vi "configuration UI.vi"() -> ()   [LabVIEW 2015, in "TDMS datalogger editor node.lvclass"]
uses:
  TDMS datalogger editor node.lvclass
  <vilib>/NI/Configuration Framework/Node/NodeRef.ctl
  <vilib>/NI/Configuration Framework/Node/NISE_CEF_Node.lvclass
  <vilib>/NI/AMC/Message Queue.ctl
  <vilib>/NI/AMC/Message.ctl
  <vilib>/NI/Tools/Keyed Array/KeyedArray.ctl
  <vilib>/NI/Configuration Framework/Node/UserEventRef.ctl
  <vilib>/NI/Configuration Framework/Controls/EventCluster.ctl
  <vilib>/NI/DCAF UI Toolkit/Controls/Move One Right.ctl
  <vilib>/NI/DCAF UI Toolkit/Controls/Move All Right.ctl
  <vilib>/NI/DCAF UI Toolkit/Controls/Move One Left.ctl
  <vilib>/NI/Configuration Framework/Node/NodeChangeEvent.ctl
  module/configuration/Logging Type.ctl
  module/configuration/Edge Direction.ctl
  module/configuration/Trigger Type.ctl
  module/configuration/Hidable controls.ctl
  module/configuration/TDMS datalogger configuration.lvclass
  <vilib>/Utility/miscctls.llb/LVPositionTypeDef.ctl
  TDMS datalogger editor node.lvclass/TDMS datalogger editor node.ctl
  module/configuration/TDMS datalogger configuration.lvclass/TDMS datalogger configuration.ctl
  <vilib>/NI/Tag Bus/tag/tag descriptor.lvclass/tag descriptor.ctl
  <vilib>/NI/Configuration Framework/serializable configuration/NISE_CEF_serializable configuration.lvclass/NISE_CEF_serializable configuration.ctl
  module/configuration/Write scans per write.vi
  module/configuration/Write queue size.vi
  module/configuration/Write Pre-trigger Blocks.vi
  module/configuration/Write Blocks to Log.vi
  module/configuration/Write Path.vi
  module/configuration/Write log name.vi
  module/configuration/Write backup directory.vi
  module/configuration/Read logrotate_options.vi
  module/configuration/Write logrotate_options.vi
  module/configuration/Write channel pattern matches.vi
  module/configuration/Write Logging Type.vi
  module/configuration/Write Edge Direction.vi
  module/configuration/Write Trigger Type.vi
  Write channel table.vi
  Write avail tags table.vi
  module/configuration/Read backup directory.vi
  module/configuration/Read Path.vi
  module/configuration/Read queue size.vi
  module/configuration/Read scans per write.vi
  module/configuration/Read add enable channel.vi
  module/configuration/Read channel pattern matches.vi
  module/configuration/Read log name.vi
  module/configuration/Read Trigger Type.vi
  module/configuration/Read Pre-trigger Blocks.vi
  module/configuration/Read Logging Type.vi
  module/configuration/Read Edge Direction.vi
  module/configuration/Read Blocks to Log.vi
  <vilib>/NI/DCAF/Tag Editor Core/Configuration Editor/Classes/Module editor node/Read Module Configuration.vi
  <vilib>/Utility/LVClass/Get LV Class Name.vi
  <vilib>/NI/Configuration Framework/error generator/NISE_error generator.vi
  Table Items.vi
  <vilib>/NI/Tag Bus Module Framework/module configuration/TBM module configuration.lvclass
  <vilib>/NI/Tag Bus/tag/tag descriptor.lvclass
  <vilib>/NI/DCAF/Tag Editor Core/Configuration Editor/Classes/Module editor node/module editor node.lvclass
  <vilib>/NI/Module Execution Interface/Engine Configuration/engine configuration.lvclass
  <vilib>/NI/Configuration Framework/NISE_CEF_TreeControl.lvlib
  <vilib>/NI/DCAF/Tag Editor Core/Configuration Editor/Classes/Engine Parent/Engine Parent Editor Node.lvclass
  <vilib>/NI/Configuration Framework/serializable configuration/NISE_CEF_serializable configuration.lvclass
  <vilib>/NI/DCAF UI Toolkit/Controls/DCAF UI Elements.lvlib
  <vilib>/NI/Tools/Keyed Array/Tools_KeyedArray.lvlib
  <vilib>/NI/AMC/AMC.lvlib
panel:
  in  "output cluster":T1
  in  "node change":T2
  in  "Tab Control":T3(tab)
  in  "Filter":string
  in  "channels":i32(listbox)
  in  "remove":T4
  in  "avail tags":i32(listbox)=-1
  in  "add all":T5
  in  "add1":T6
  in  "Edge Direction":T7
  out "Trigger Channel":string
  in  "Trigger Type":T8
  in  "Total Blocks to Log":i32=20
  in  "Pre-trigger Blocks":i32=20
  in  "Logging Type":T9
  out "Enable Tag":string
  in  "use enable channel":bool
  in  "queue size":u16=2
  in  "file name error":bool
  in  "Log Directory":string
  in  "File Name":string
  in  "path error":bool
  in  "recalc":bool
  out "Approximate memory usage":dbl
  in  "Block Size (scans per write)":u16=20
  in  "Log Directory":path
  in  "Maximum age of files (days)":dbl=365.0
  in  "Maximum file size (KB)":i64=10000
  in  "Rotate count":u32 caption="Maximum number of archived files to keep"
  in  "archive in place":bool caption="Archive old logs in original directory"
  in  "Archive Directory":string
  in  "Archive Directory":path
  in  "archive error":bool
  in  "Channel Subscription Pattern Matches":string[](array[string])
  in  "Enable Dynamic Mapping":bool
  in  "user event":T10
  in  "main queue":T11
  in  "node ref":T12
  # "Note: This value ignores dynamic mapping"
  # "kB"
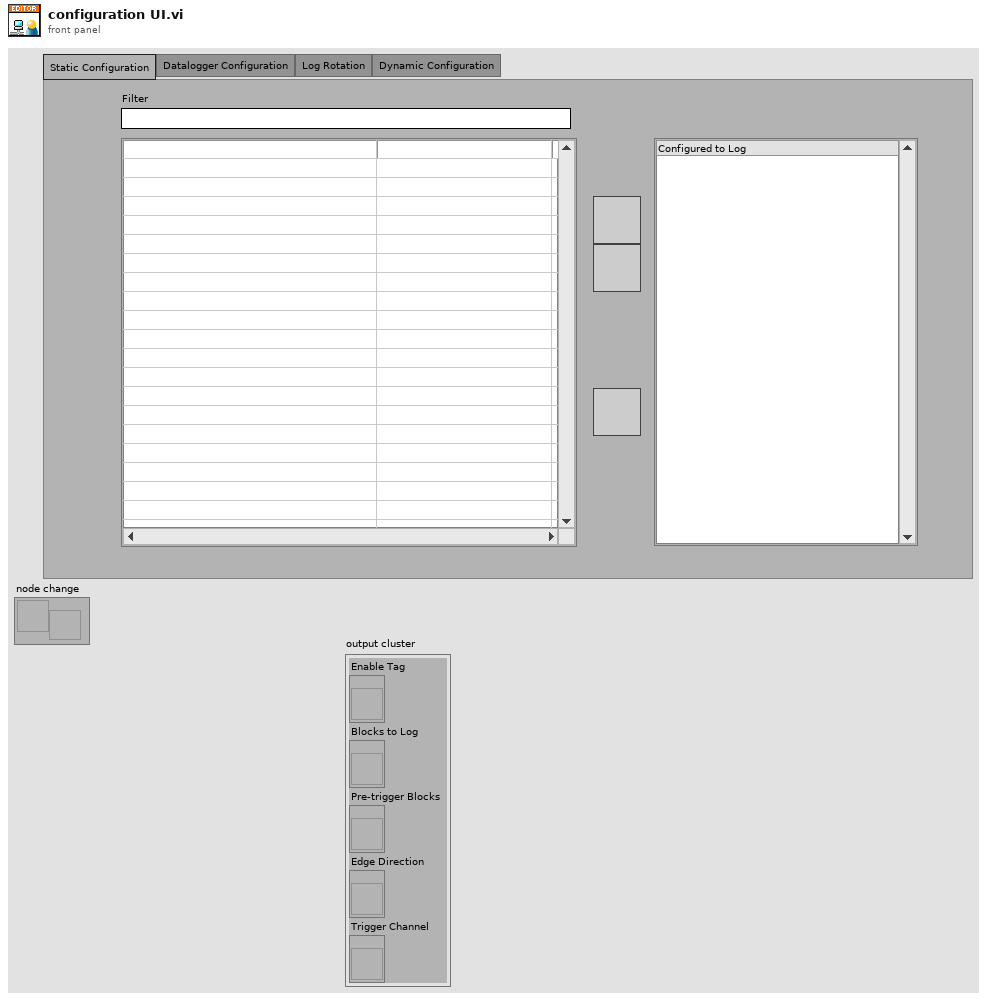
[diagram p1: front panel]
types:
  T1 = typedef "TDMS datalogger editor node.lvclass/Hidable controls.ctl" = cluster{"Enable Tag":refnum<vi>, "Blocks to Log":refnum<vi>, "Pre-trigger Blocks":refnum<vi>, "Edge Direction":refnum<vi>, "Trigger Channel":refnum<vi>}
  T2 = typedef "NISE_CEF_Node.lvclass/NodeChangeEvent.ctl" = refnum<user-event>
  T3 = enum32{"Static Configuration", "Datalogger Configuration", "Log Rotation", "Dynamic Configuration"}
  T4 = typedef "DCAF UI Elements.lvlib/Move One Left.ctl" = bool
  T5 = typedef "DCAF UI Elements.lvlib/Move All Right.ctl" = bool
  T6 = typedef "DCAF UI Elements.lvlib/Move One Right.ctl" = bool
  T7 = typedef "TDMS datalogger configuration.lvclass/Edge Direction.ctl" = enum16{"Rising", "Falling"}
  T8 = typedef "TDMS datalogger configuration.lvclass/Trigger Type.ctl" = enum16{"None", "Start"}
  T9 = typedef "TDMS datalogger configuration.lvclass/Logging Type.ctl" = enum16{"Continuous", "Finite"}
  T10 = typedef "NISE_CEF_Node.lvclass/UserEventRef.ctl" = refnum<user-event>
  T11 = typedef "AMC.lvlib/Message Queue.ctl" = refnum<queue>
  T12 = typedef "NISE_CEF_Node.lvclass/NodeRef.ctl" = refnum<data-value>
  T13 = typedef "LVPositionTypeDef.ctl" = cluster{"Left":i32, "Top":i32}
  T14 = typedef "NISE_CEF_TreeControl.lvlib/EventCluster.ctl" = cluster{"command":string, "data":string}
  T15 = typedef "TBM configuration.lvclass/Target Types.ctl" = enum16{"Windows", "Mac", "Linux", "Linux RT ARM", "VxWorks", "Pharlap", "Other", "Linux RT x64"}
  T16 = typedef "LogRotate.lvclass/options.ctl" = cluster{"max file size (bytes)":i64, "rotate count":u32, "max age (days)":dbl, "No archive dir":bool, "Archive dir":path}
  T17 = typedef "tag bus.lvlib/tag descriptor.lvclass/Data Type.ctl" = enum16{"Double", "Single", "I64", "I32", "I16", "I8", "U64", "U32", "U16", "U8", "Boolean", "String", "Array of Double", "Array of Single", "Array of I64", "Array of I32", "Array of I16", "Array of I8", "Array of U64", "Array of U32", "Array of U16", "Array of U8", "Array of Boolean", "Array of String"}
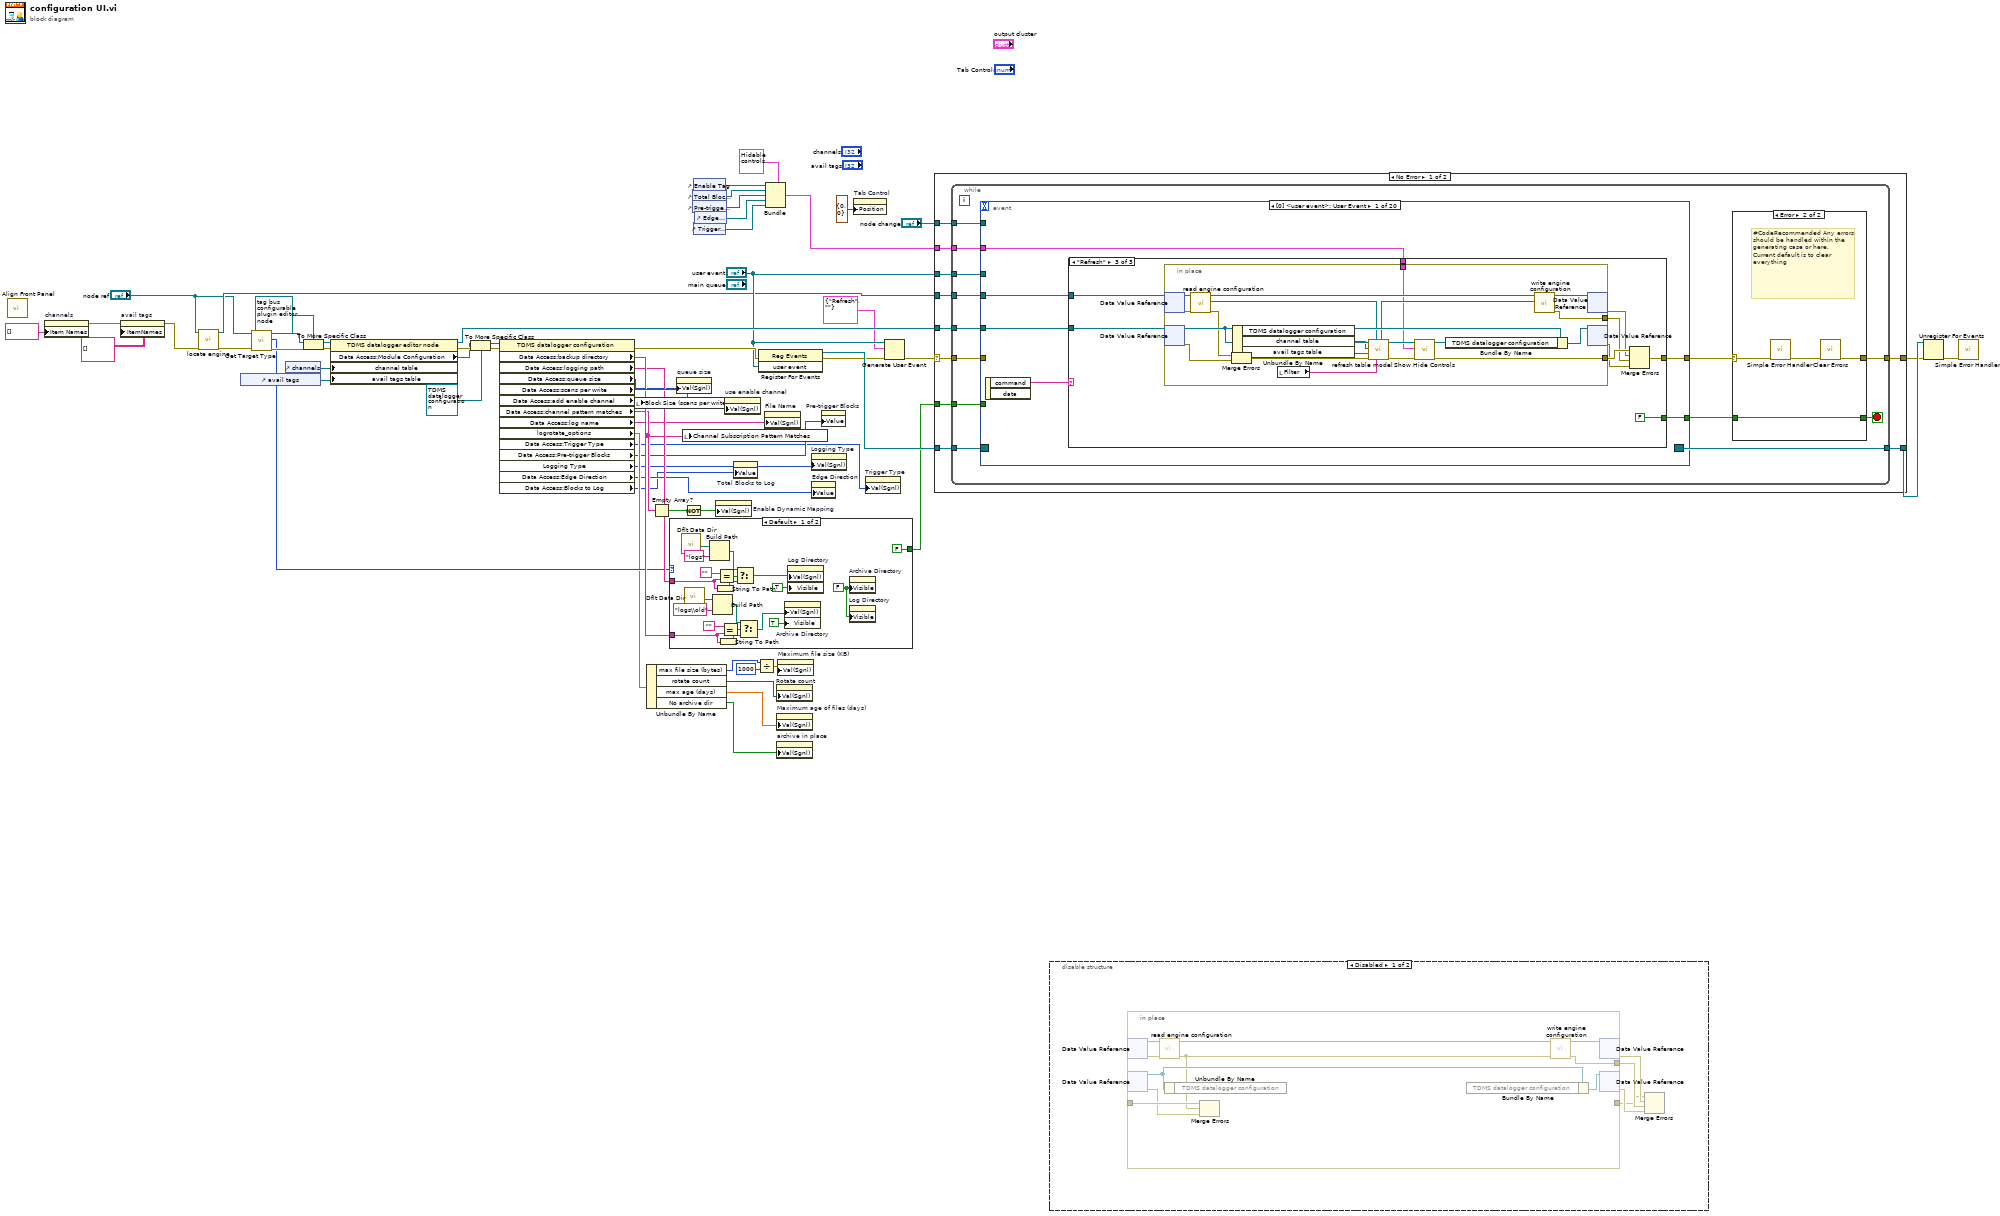
[diagram p0: block diagram]
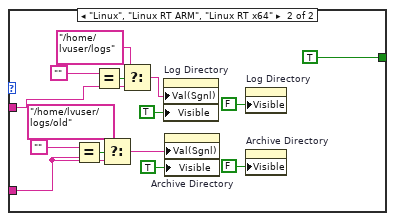
[diagram p2: hidden frame]
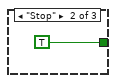
[diagram p5: hidden frame]
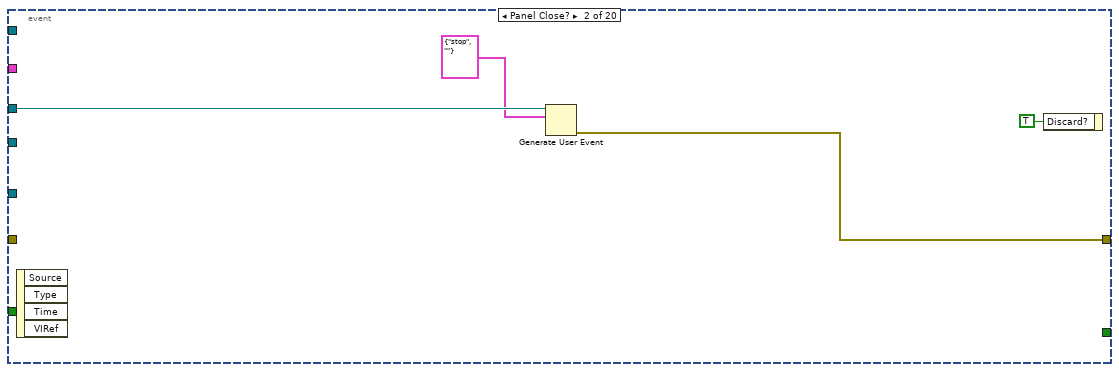
[diagram p6: hidden frame]
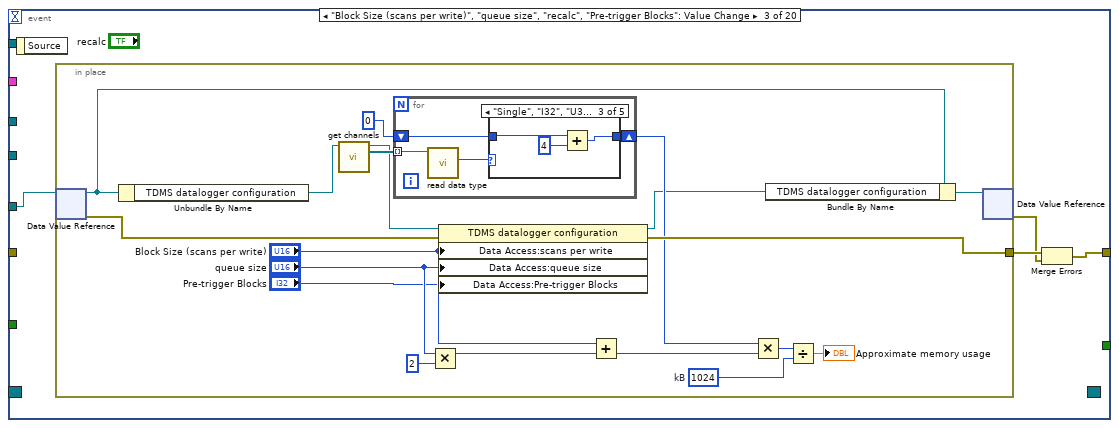
[diagram p7: hidden frame]
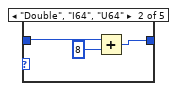
[diagram p9: hidden frame]
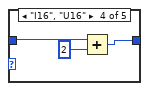
[diagram p10: hidden frame]
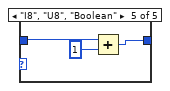
[diagram p11: hidden frame]
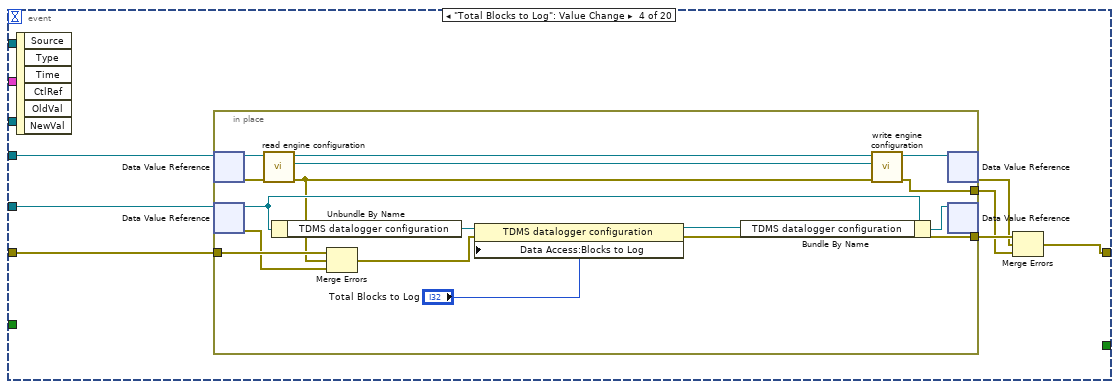
[diagram p12: hidden frame]
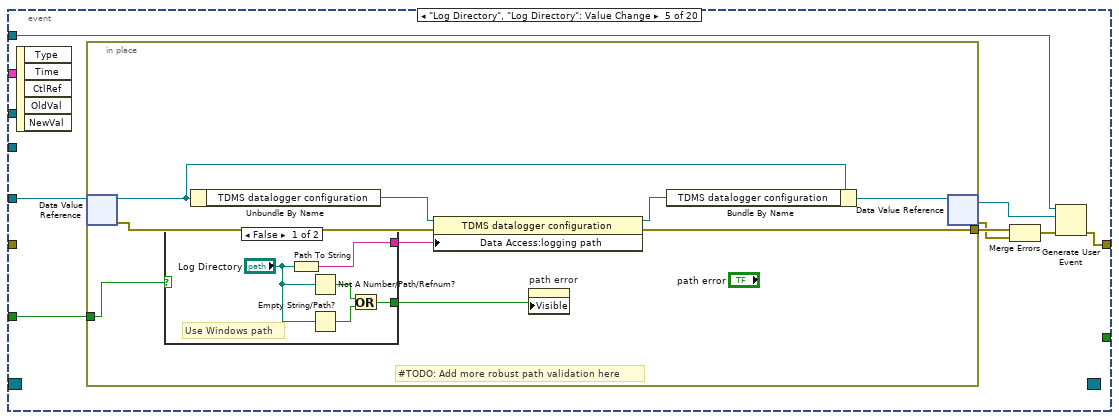
[diagram p13: hidden frame]
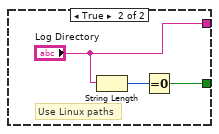
[diagram p14: hidden frame]
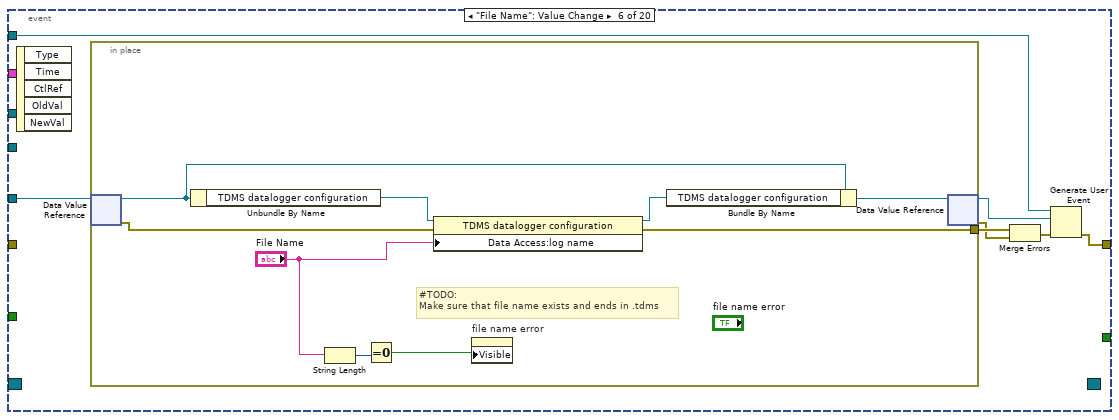
[diagram p15: hidden frame]
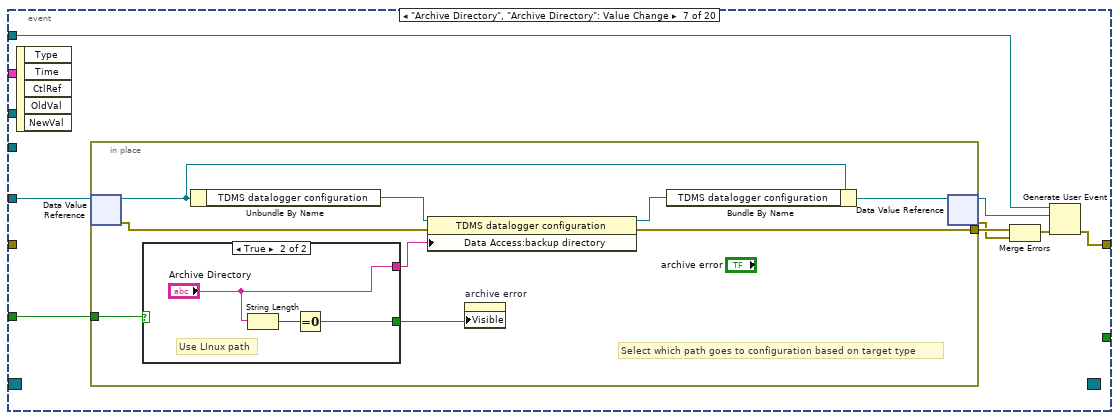
[diagram p16: hidden frame]
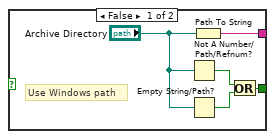
[diagram p17: hidden frame]
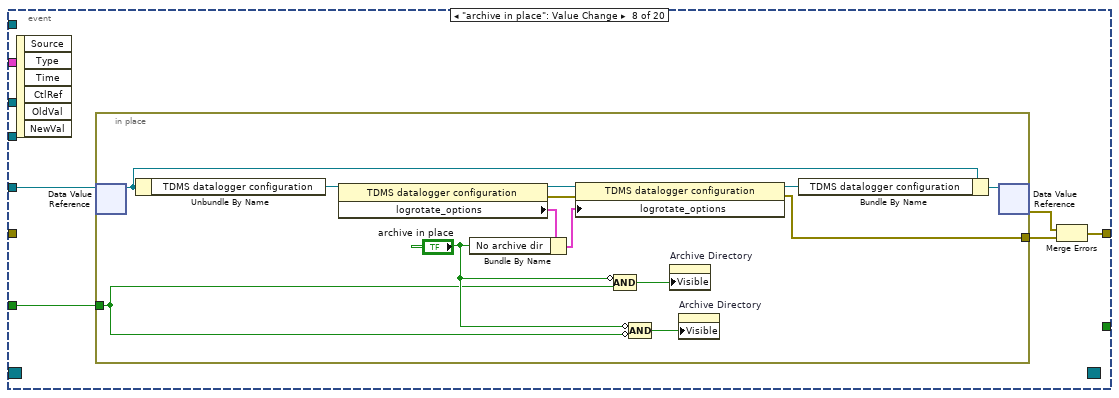
[diagram p18: hidden frame]
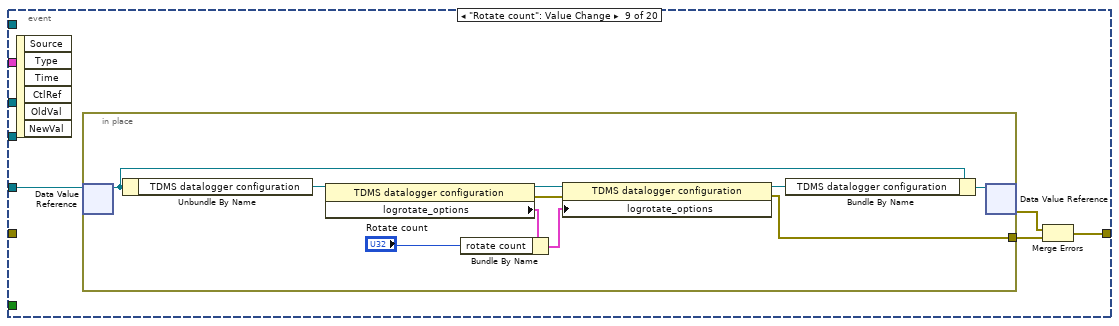
[diagram p19: hidden frame]
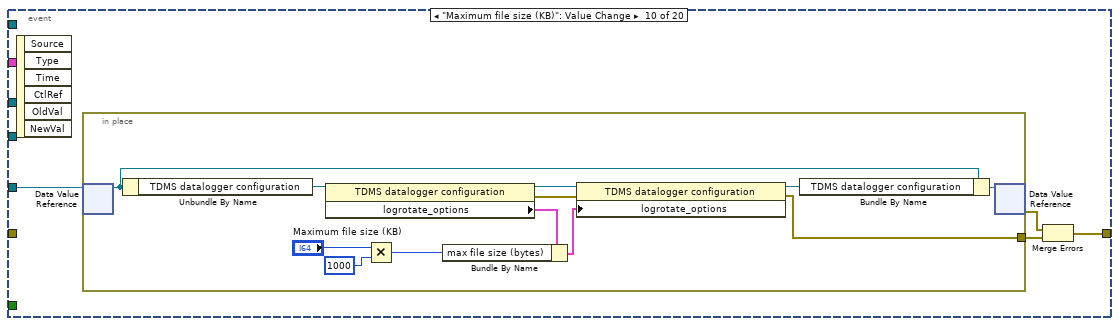
[diagram p20: hidden frame]
diagram:
  n1 = call <vilib>:"Align Front Panel.vi"() -> ()  [unwired: 10 in, 2 out]
  n2 = property on="channels" class="LstBox (strict)"("Item Names"=string[] []) -> (error out=w44:errorcluster)  [unwired: 2 in, 1 out]
  n3 = property on="avail tags" class="MCListbox (strict)"(error in=w44, "ItemNames"=string[][] [] ("Item Names")) -> (error out=w36:errorcluster)  [unwired: 1 in, 1 out]
  n4 = call <vilib>:"locate engine.vi"("error in"=w36, "component"="node ref") -> ("error out"=w26:errorcluster, "engine"=w35:refnum<data-value>)  [unwired: 8 in]
  n5 = control-ref of="avail tags"() -> (w20:refnum<vi>)
  n6 = call "Get Target Type.vi"("error in (no error)"=w26, "node ref in"="node ref") -> ("error out"=w29:errorcluster, "Target Type"=w25:T15, "node ref out"=w28:T12)  [unwired: 6 in]
  n7 = control-ref of="channels"() -> (w21:refnum<vi>)
  n8 = To More Specific Class(target class=refnum<data-value> refnum ("data value reference"), reference=w28, error in=w29) -> (specific class reference=w38:refnum<data-value>, error out=w37:errorcluster)
  n9 = property class="TDMS datalogger editor node"(reference=w38, error in=w37, "channel table"=w21, "avail tags table"=w20) -> (reference out=w40:refnum<data-value>, error out=w58:errorcluster, "Data Access:Module Configuration"=w48:refnum<class "TBM module configuration.lvclass">)
  n10 = To More Specific Class(target class=refnum<class "TDMS datalogger configuration.lvclass"> refnum ("TDMS datalogger configuration"), reference=w48, error in=w58) -> (specific class reference=w46:refnum<class "TDMS datalogger configuration.lvclass">, error out=w49:errorcluster)
  n11 = property class="TDMS datalogger configuration"(reference=w46, error in=w49) -> (error out=w45:errorcluster, "Data Access:backup directory"=w55:string, "Data Access:logging path"=w54:string, "Data Access:queue size"=w53:u16, "Data Access:scans per write"=w57:u16, "Data Access:add enable channel"=w56:bool, "Data Access:channel pattern matches"=w52:string[], "Data Access:log name"=w24:string, "logrotate_options"=w19:T16, "Data Access:Trigger Type"=w3:T8, "Data Access:Pre-trigger Blocks"=w4:i32, "Logging Type"=w1:T9, "Data Access:Edge Direction"=w5:T7, "Data Access:Blocks to Log"=w2:i32)  [unwired: 1 out]
  n12 = local write "Block Size (scans per write)"(w57) -> ()
  n13 = Unbundle By Name(w19) -> ("max file size (bytes)"=w15:i64, "rotate count"=w17:u32, "max age (days)"=w18:dbl, "No archive dir"=w16:bool)
  n14 = Empty Array?(array=w52) -> (empty?=w50:bool)
  n15 = case shown="Default" w25 {
    tunnel: w55 -> [w63 w82]
    tunnel: w54 -> [w72 w89]
    tunnel: [FALSE TRUE] -> w23
    frame Default {
      w79 = FALSE ("Visible")
      n16 = call <vilib>:"Dflt Data Dir.vi"() -> ("App:Default Data Directory"=w75:path)
      n17 = call <vilib>:"Dflt Data Dir.vi"() -> ("App:Default Data Directory"=w66:path)
      n18 = Build Path(base path=w75, name or relative path="logs") -> (appended path=w77:path)
      n19 = Build Path(base path=w66, name or relative path="logs\\old") -> (appended path=w64:path)
      n20 = String To Path(string=w72) -> (path=w71:path)
      n21 = Equal?(x="", y=w72) -> (x = y?=w73:bool)
      n22 = String To Path(string=w63) -> (path=w69:path)
      n23 = Equal?(x="", y=w63) -> (x = y?=w68:bool)
      n24 = Select(t=w77, s=w73, f=w71) -> (s? t:f=w70:path)
      n25 = Select(t=w64, s=w68, f=w69) -> (s? t:f=w62:path)
      n26 = property on="Archive Directory" class="Path"("Val(Sgnl)"=w62, "Visible"=TRUE) -> ()  [unwired: 2 in, 2 out]
      n27 = property on="Log Directory" class="Path"("Val(Sgnl)"=w70, "Visible"=TRUE) -> ()  [unwired: 2 in, 2 out]
      n28 = property on="Archive Directory" class="Str"("Visible"=w79) -> ()  [unwired: 2 in, 2 out]
      n29 = property on="Log Directory" class="Str"("Visible"=w79) -> ()  [unwired: 2 in, 2 out]
    }
    frame "Linux", "Linux RT ARM", "Linux RT x64" {
      n30 = Equal?(x="", y=w82) -> (x = y?=w85:bool)
      n31 = Equal?(x="", y=w89) -> (x = y?=w90:bool)
      n32 = Select(t="/home/lvuser/logs/old", s=w85, f=w82) -> (s? t:f=w83:string)
      n33 = Select(t="/home/lvuser/logs", s=w90, f=w89) -> (s? t:f=w88:string)
      n34 = property on="Log Directory" class="Str"("Val(Sgnl)"=w88, "Visible"=TRUE) -> ()  [unwired: 2 in, 2 out]
      n35 = property on="Archive Directory" class="Str"("Val(Sgnl)"=w83, "Visible"=TRUE) -> ()  [unwired: 2 in, 2 out]
      n36 = property on="Log Directory" class="Path"("Visible"=FALSE) -> ()  [unwired: 2 in, 2 out]
      n37 = property on="Archive Directory" class="Path"("Visible"=FALSE) -> ()  [unwired: 2 in, 2 out]
    }
  }
  n38 = property on="queue size" class="DigNum (strict)"("Val(Sgnl)"=w53) -> ()  [unwired: 2 in, 2 out]
  n39 = local write "Channel Subscription Pattern Matches"(w52) -> ()
  n40 = Not(x=w50) -> (.not. x?=w51:bool)
  n41 = control-ref of="Total Blocks to Log"() -> (w8:refnum<vi>)
  n42 = control-ref of="Pre-trigger Blocks"() -> (w11:refnum<vi>)
  n43 = control-ref of="Enable Tag"() -> (w12:refnum<vi>)
  n44 = control-ref of="Trigger Channel"() -> (w6:refnum<vi>)
  n45 = control-ref of="Edge Direction"() -> (w7:refnum<vi>)
  n46 = property on="Enable Dynamic Mapping" class="Bool (strict)"("Val(Sgnl)"=w51) -> ()  [unwired: 2 in, 2 out]
  n47 = property on="use enable channel" class="Bool (strict)"("Val(Sgnl)"=w56) -> ()  [unwired: 2 in, 2 out]
  n48 = property on="Total Blocks to Log" class="DigNum (strict)"("Value"=w2) -> ()  [unwired: 2 in, 2 out]
  n49 = Divide(x=w15, y=i64 1000) -> (x/y=w14:dbl)
  n50 = register-events(error in=w45, "user event") -> (reference out=w61:refnum<event-registration>, error out=w33:errorcluster)  [unwired: 1 in]
  n51 = property on="File Name" class="Str"("Val(Sgnl)"=w24) -> ()  [unwired: 2 in, 2 out]
  n52 = Bundle(cluster=T1 {"Enable Tag"=refnum, "Blocks to Log"=refnum, "Pre-trigger Blocks"=refnum, "Edge Direction"=refnum, "Trigger Channel"=refnum} ("output cluster"), "Enable Tag"=w12, "Blocks to Log"=w8, "Pre-trigger Blocks"=w11, "Edge Direction"=w7, "Trigger Channel"=w6) -> (w9:T1)
  n53 = property on="Rotate count" class="DigNum (strict)"("Val(Sgnl)"=w17) -> ()  [unwired: 2 in, 2 out]
  n54 = property on="Maximum age of files (days)" class="DigNum (strict)"("Val(Sgnl)"=w18) -> ()  [unwired: 2 in, 2 out]
  n55 = property on="archive in place" class="Bool (strict)"("Val(Sgnl)"=w16) -> ()  [unwired: 2 in, 2 out]
  n56 = property on="Maximum file size (KB)" class="DigNum (strict)"("Val(Sgnl)"=w14) -> ()  [unwired: 2 in, 2 out]
  n57 = property on="Logging Type" class="Enum (strict)"("Val(Sgnl)"=w1) -> ()  [unwired: 2 in, 2 out]
  n58 = property on="Edge Direction" class="Enum (strict)"("Value"=w5) -> ()  [unwired: 2 in, 2 out]
  n59 = property on="Pre-trigger Blocks" class="DigNum (strict)"("Value"=w4) -> ()  [unwired: 2 in, 2 out]
  n60 = property on="Tab Control" class="TabCtl (strict)"("Position"=T13 {"Left"=0, "Top"=0}) -> ()  [unwired: 2 in, 2 out]
  n61 = property on="Trigger Type" class="Enum (strict)"("Val(Sgnl)"=w3) -> ()  [unwired: 2 in, 2 out]
  n62 = Generate User Event(user event="user event", event data cluster=T14 {"command"="Refresh", "data"=""} ("event data"), error in=w33) -> (error out=w32:errorcluster)  [unwired: 1 in, 1 out]
  n63 = case shown="No Error" w32 {
    selector: w32 -> [w97 w614]
    tunnel: w61 -> [w106 w613]
    tunnel: [w105 w613] -> w60
    tunnel: [w104 w614] -> w41
    tunnel: w40 -> [w103 _]
    tunnel: w35 -> [w102 _]
    tunnel: "user event" -> [w101 _]
    tunnel: w23 -> [w100 _]
    tunnel: "node change" -> [w99 _]
    tunnel: w9 -> [w98 _]
    frame No Error {
      n64 = while {
        tunnel: w106 -> [w119]
        tunnel: [w118] -> w105
        tunnel: w102 -> [w114]
        tunnel: w103 -> [w113]
        tunnel: w101 -> [w112]
        tunnel: [w115] -> w104
        tunnel: w100 -> [w110]
        tunnel: w99 -> [w109]
        tunnel: w98 -> [w108]
        tunnel: w97 -> [w107]
        stop <- w116 stop-if-true
        n65 = event shown="[0] <user event>: User Event" {
          selector: w119 -> [_ _ _ _ _ _ _ _ _ _ _ _ _ _ _ _ _ _ _ _]
          dyn-events: [_ _ _ _ _ _ _ _ _ _ _ _ _ _ _ _ _ _ _ _] -> w118
          timeout: _ -> [_ _ _ _ _ _ _ _ _ _ _ _ _ _ _ _ _ _ _ _]
          tunnel: [w131 _ _ _ _ _ _ _ _ _ _ _ _ _ _ _ _ _ _ _] -> w111
          tunnel: [w129 w165 w168 w209 w232 w255 w273 w299 w316 w330 w346 w358 w381 w437 w467 w503 w540 w560 w572 w604] -> w117
          tunnel: w114 -> [w128 _ _ w211 _ _ _ _ _ _ _ _ w379 w438 w465 w498 _ _ w570 _]
          tunnel: w113 -> [w127 _ w169 w212 w236 w260 w277 w300 w317 w331 w347 w359 w380 w439 w466 w499 w542 w562 w571 _]
          tunnel: w112 -> [_ w164 _ _ _ _ _ _ _ _ _ _ w383 w444 w472 w500 w543 _ w578 _]
          tunnel: w110 -> [_ _ _ _ w234 _ w275 w296 _ _ _ _ _ _ _ _ _ _ _ _]
          tunnel: w109 -> [_ _ _ _ w230 w258 w272 _ _ _ _ _ _ _ _ _ _ _ _ _]
          tunnel: w108 -> [w126 _ _ _ _ _ _ _ _ _ _ _ _ _ _ _ _ _ _ _]
          tunnel: w107 -> [_ _ _ w213 _ _ _ _ _ _ _ _ _ _ _ _ _ _ _ w603]
          event User Event {
            n66 = event-data() -> ("command"=w130:string)  [unwired: 1 in, 1 out]
            n67 = case shown="\"Refresh\"" w130 {
              tunnel: [_ TRUE FALSE] -> w131
              tunnel: [_ _ w139] -> w129
              tunnel: w128 -> [_ _ w138]
              tunnel: w127 -> [_ _ w137]
              tunnel: w126 -> [_ _ w133]
              frame Default {
              }
              frame "Stop" {
              }
              frame "Refresh" {
                n68 = in-place {
                  in-place-border: [w146] -> w140
                  in-place-border: [w150] -> w136
                  in-place-border: w133 -> [w143]
                  n69 = in-place-dvr #1(w138) -> (w154:refnum<class "Engine Parent Editor Node.lvclass">, w155:errorcluster)
                  n70 = in-place-dvr #2(w137) -> (w160:refnum<class "TDMS datalogger editor node.lvclass">, w158:errorcluster)
                  n71 = call <vilib>:"read engine configuration.vi"("error in"=w155, "Engine Parent Editor Node in"=w154) -> ("error out"=w151:errorcluster, "engine configuration"=w152:refnum<class "engine configuration.lvclass">, "Engine Parent Editor Node out"=w153:refnum<class "Engine Parent Editor Node.lvclass">)  [unwired: 7 in]
                  n72 = Merge Errors(w151, w158) -> (w162:errorcluster)
                  n73 = Unbundle By Name(w160) -> ("TDMS datalogger configuration"=w161:refnum<class "TDMS datalogger configuration.lvclass">, "channel table"=w149:refnum<vi>, "avail tags table"=w148:refnum<vi>)
                  n74 = local read "Filter"() -> (w142:string)
                  n75 = call "refresh table model.vi"("Filter"=w142, "engine configuration"=w152, "error in"=w162, "avail tags"=w148, "chan table"=w149, "TDMS datalogger configuration"=w161) -> ("error out"=w147:errorcluster, "TDMS datalogger configuration out"=w144:refnum<class "TDMS datalogger configuration.lvclass">, "engine configuration out"=w156:refnum<class "engine configuration.lvclass">)  [unwired: 3 in]
                  n76 = call "Show Hide Controls.vi"("error in (no error)"=w147, "Hidable Controls"=w143, "TDMS datalogger configuration"=w144) -> ("error out"=w146:errorcluster, "Datalogger configuration out"=w145:refnum<class "TDMS datalogger configuration.lvclass">)  [unwired: 7 in]
                  n77 = Bundle By Name(cluster=w160, "TDMS datalogger configuration"=w145) -> (w159:refnum<class "TDMS datalogger editor node.lvclass">)
                  n78 = call <vilib>:"write engine configuration.vi"("engine configuration"=w156, "Engine Parent Editor Node in"=w153) -> ("error out"=w150:errorcluster, "Engine Parent Editor Node out"=w157:refnum<class "Engine Parent Editor Node.lvclass">)  [unwired: 8 in]
                  n79 = in-place-dvr #1(w157) -> (w135:errorcluster)  [unwired: 1 out]
                  n80 = in-place-dvr #2(w159) -> (w134:errorcluster)  [unwired: 1 out]
                }
                n81 = Merge Errors(w140, w135, w136, w134) -> (w139:errorcluster)
              }
            }
          }
          event Panel Close? {
            n82 = event-data() -> ()  [unwired: 1 in, 4 out]
            n83 = Generate User Event(user event=w164, event data cluster=T14 {"command"="stop", "data"=""} ("event data")) -> (error out=w165:errorcluster)  [unwired: 2 in, 1 out]
            n84 = event-data("Discard?"=TRUE) -> ()  [unwired: 1 in, 1 out]
          }
          event "Block Size (scans per write)", "queue size", "recalc", "Pre-trigger Blocks": Value Change {
            n85 = event-data() -> ()  [unwired: 1 in, 1 out]
            n86 = in-place {
              in-place-border: [w189] -> w170
              w186 = u32 1024  # kB
              n87 = in-place-dvr #3(w169) -> (w179:refnum<class "TDMS datalogger editor node.lvclass">, w180:errorcluster)
              n88 = Unbundle By Name(w179) -> ("TDMS datalogger configuration"=w177:refnum<class "TDMS datalogger configuration.lvclass">)
              n89 = call-dynamic "get channels.vi"("module configuration in"=w177) -> ("channels"=w183:refnum<class "TBM channel.lvclass">[], "module configuration out"=w181:refnum<class "TDMS datalogger configuration.lvclass">)  [unwired: 9 in]
              n90 = for {
                shift-right: [w192] -> w184
                shift-left: u32 0 -> [w193]
                tunnel: w183 -> [w190] mode=indexing
                n91 = call <vilib>:"read data type.vi"("system tag in"=w190) -> ("data type"=w191:T17)  [unwired: 8 in, 2 out]
                n92 = case shown="\"Single\", \"I32\", \"U32\"" w191 {
                  tunnel: w193 -> [w194 w197 w200 w203 w206]
                  tunnel: [w194 w196 w199 w202 w205] -> w192
                  frame Default {
                  }
                  frame "Double", "I64", "U64" {
                    n93 = Add(x=w197, y=u32 8) -> (x+y=w196:u32)
                  }
                  frame "Single", "I32", "U32" {
                    n94 = Add(x=w200, y=u32 4) -> (x+y=w199:u32)
                  }
                  frame "I16", "U16" {
                    n95 = Add(x=w203, y=u32 2) -> (x+y=w202:u32)
                  }
                  frame "I8", "U8", "Boolean" {
                    n96 = Add(x=w206, y=u32 1) -> (x+y=w205:u32)
                  }
                }
              }
              n97 = Multiply(x="queue size", y=2 ("x")) -> (x*y=w173:i32)
              n98 = property class="TDMS datalogger configuration"(reference=w181, error in=w180, "Data Access:scans per write"="Block Size (scans per write)", "Data Access:queue size"="queue size", "Data Access:Pre-trigger Blocks"="Pre-trigger Blocks") -> (reference out=w176:refnum<class "TDMS datalogger configuration.lvclass">, error out=w189:errorcluster)
              n99 = Add(x="Block Size (scans per write)", y=w173) -> (x+y=w174:i32)
              n100 = Multiply(x=w184, y=w174) -> (x*y=w175:u32)
              n101 = Bundle By Name(cluster=w179, "TDMS datalogger configuration"=w176) -> (w178:refnum<class "TDMS datalogger editor node.lvclass">)
              n102 = Divide(x=w175, y=w186) -> (x/y=→"Approximate memory usage":dbl)
              n103 = in-place-dvr #3(w178) -> (w167:errorcluster)  [unwired: 1 out]
            }
            n104 = Merge Errors(w170, w167) -> (w168:errorcluster)
          }
          event "Total Blocks to Log": Value Change {
            n105 = event-data() -> ()  [unwired: 1 in, 6 out]
            n106 = in-place {
              in-place-border: w213 -> [w229]
              in-place-border: [w222] -> w207
              in-place-border: [w215] -> w210
              n107 = in-place-dvr #4(w211) -> (w224:refnum<class "Engine Parent Editor Node.lvclass">, w225:errorcluster)
              n108 = in-place-dvr #5(w212) -> (w221:refnum<class "TDMS datalogger editor node.lvclass">, w227:errorcluster)
              n109 = call <vilib>:"read engine configuration.vi"("error in"=w225, "Engine Parent Editor Node in"=w224) -> ("error out"=w220:errorcluster, "engine configuration"=w214:refnum<class "engine configuration.lvclass">, "Engine Parent Editor Node out"=w223:refnum<class "Engine Parent Editor Node.lvclass">)  [unwired: 7 in]
              n110 = Unbundle By Name(w221) -> ("TDMS datalogger configuration"=w219:refnum<class "TDMS datalogger configuration.lvclass">)
              n111 = Merge Errors(w229, w220, w227) -> (w217:errorcluster)
              n112 = property class="TDMS datalogger configuration"(reference=w219, error in=w217, "Data Access:Blocks to Log"="Total Blocks to Log") -> (reference out=w218:refnum<class "TDMS datalogger configuration.lvclass">, error out=w215:errorcluster)
              n113 = Bundle By Name(cluster=w221, "TDMS datalogger configuration"=w218) -> (w228:refnum<class "TDMS datalogger editor node.lvclass">)
              n114 = call <vilib>:"write engine configuration.vi"("error in"=w220, "engine configuration"=w214, "Engine Parent Editor Node in"=w223) -> ("error out"=w222:errorcluster, "Engine Parent Editor Node out"=w226:refnum<class "Engine Parent Editor Node.lvclass">)  [unwired: 7 in]
              n115 = in-place-dvr #4(w226) -> (w208:errorcluster)  [unwired: 1 out]
              n116 = in-place-dvr #5(w228) -> ()  [unwired: 2 out]
            }
            n117 = Merge Errors(w210, w208, w207) -> (w209:errorcluster)
          }
          event "Log Directory", "Log Directory": Value Change {
            n118 = event-data() -> ()  [unwired: 1 in, 5 out]
            n119 = in-place {
              in-place-border: [w246] -> w237
              in-place-border: w234 -> [w238]
              # "#TODO: Add more robust path validation here"
              n120 = in-place-dvr #6(w236) -> (w240:refnum<class "TDMS datalogger editor node.lvclass">, w243:errorcluster)
              n121 = case shown="False" w238 {
                tunnel: [w248 w252] -> w245
                tunnel: [w247 "Log Directory"] -> w239
                frame False {
                  # "Use Windows path"
                  n122 = Path To String(path="Log Directory") -> (string=w247:string)
                  n123 = Not A Number/Path/Refnum?(number/path/refnum="Log Directory") -> (NaN/Path/Refnum?=w249:bool)
                  n124 = Empty String/Path?(string/path="Log Directory") -> (empty?=w250:bool)
                  n125 = Or(x=w249, y=w250) -> (x .or. y?=w248:bool)
                }
                frame True {
                  # "Use Linux paths"
                  n126 = String Length(string="Log Directory") -> (length=w253:i32)
                  n127 = Equal To 0?(x=w253) -> (x = 0?=w252:bool)
                }
              }
              n128 = Unbundle By Name(w240) -> ("TDMS datalogger configuration"=w244:refnum<class "TDMS datalogger configuration.lvclass">)
              n129 = property class="TDMS datalogger configuration"(reference=w244, error in=w243, "Data Access:logging path"=w239) -> (reference out=w242:refnum<class "TDMS datalogger configuration.lvclass">, error out=w246:errorcluster)
              n130 = property on="path error" class="Bool"("Visible"=w245) -> ()  [unwired: 2 in, 2 out]
              n131 = Bundle By Name(cluster=w240, "TDMS datalogger configuration"=w242) -> (w241:refnum<class "TDMS datalogger editor node.lvclass">)
              n132 = in-place-dvr #6(w241) -> (w231:refnum<data-value>, w235:errorcluster)
            }
            n133 = Merge Errors(w237, w235) -> (w233:errorcluster)
            n134 = Generate User Event(user event=w230, event data cluster=w231, error in=w233) -> (error out=w232:errorcluster)  [unwired: 1 in, 1 out]
          }
          event "File Name": Value Change {
            n135 = event-data() -> ()  [unwired: 1 in, 5 out]
            n136 = in-place {
              in-place-border: [w270] -> w261
              # "#TODO:\nMake sure that file name exists and ends in .tdms"
              n137 = in-place-dvr #7(w260) -> (w265:refnum<class "TDMS datalogger editor node.lvclass">, w268:errorcluster)
              n138 = Unbundle By Name(w265) -> ("TDMS datalogger configuration"=w269:refnum<class "TDMS datalogger configuration.lvclass">)
              n139 = String Length(string="File Name") -> (length=w263:i32)
              n140 = Equal To 0?(x=w263) -> (x = 0?=w262:bool)
              n141 = property class="TDMS datalogger configuration"(reference=w269, error in=w268, "Data Access:log name"="File Name") -> (reference out=w267:refnum<class "TDMS datalogger configuration.lvclass">, error out=w270:errorcluster)
              n142 = property on="file name error" class="Bool"("Visible"=w262) -> ()  [unwired: 2 in, 2 out]
              n143 = Bundle By Name(cluster=w265, "TDMS datalogger configuration"=w267) -> (w266:refnum<class "TDMS datalogger editor node.lvclass">)
              n144 = in-place-dvr #7(w266) -> (w257:refnum<data-value>, w259:errorcluster)
            }
            n145 = Merge Errors(w261, w259) -> (w256:errorcluster)
            n146 = Generate User Event(user event=w258, event data cluster=w257, error in=w256) -> (error out=w255:errorcluster)  [unwired: 1 in, 1 out]
          }
          event "Archive Directory", "Archive Directory": Value Change {
            n147 = event-data() -> ()  [unwired: 1 in, 5 out]
            n148 = in-place {
              in-place-border: [w284] -> w278
              in-place-border: w275 -> [w279]
              # "Select which path goes to configuration based on target type"
              n149 = in-place-dvr #8(w277) -> (w286:refnum<class "TDMS datalogger editor node.lvclass">, w281:errorcluster)
              n150 = case shown="True" w279 {
                tunnel: [w289 w293] -> w285
                tunnel: [w288 "Archive Directory"] -> w280
                frame False {
                  # "Use Windows path"
                  n151 = Not A Number/Path/Refnum?(number/path/refnum="Archive Directory") -> (NaN/Path/Refnum?=w291:bool)
                  n152 = Empty String/Path?(string/path="Archive Directory") -> (empty?=w292:bool)
                  n153 = Path To String(path="Archive Directory") -> (string=w288:string)
                  n154 = Or(x=w291, y=w292) -> (x .or. y?=w289:bool)
                }
                frame True {
                  # "Use LInux path"
                  n155 = String Length(string="Archive Directory") -> (length=w294:i32)
                  n156 = Equal To 0?(x=w294) -> (x = 0?=w293:bool)
                }
              }
              n157 = Unbundle By Name(w286) -> ("TDMS datalogger configuration"=w282:refnum<class "TDMS datalogger configuration.lvclass">)
              n158 = property class="TDMS datalogger configuration"(reference=w282, error in=w281, "Data Access:backup directory"=w280) -> (reference out=w283:refnum<class "TDMS datalogger configuration.lvclass">, error out=w284:errorcluster)
              n159 = property on="archive error" class="Bool"("Visible"=w285) -> ()  [unwired: 2 in, 2 out]
              n160 = Bundle By Name(cluster=w286, "TDMS datalogger configuration"=w283) -> (w287:refnum<class "TDMS datalogger editor node.lvclass">)
              n161 = in-place-dvr #8(w287) -> (w271:refnum<data-value>, w276:errorcluster)
            }
            n162 = Merge Errors(w278, w276) -> (w274:errorcluster)
            n163 = Generate User Event(user event=w272, event data cluster=w271, error in=w274) -> (error out=w273:errorcluster)  [unwired: 1 in, 1 out]
          }
          event "archive in place": Value Change {
            n164 = event-data() -> ()  [unwired: 1 in, 6 out]
            n165 = in-place {
              in-place-border: [w305] -> w297
              in-place-border: w296 -> [w301]
              n166 = in-place-dvr #9(w300) -> (w308:refnum<class "TDMS datalogger editor node.lvclass">)  [unwired: 1 out]
              n167 = Unbundle By Name(w308) -> ("TDMS datalogger configuration"=w313:refnum<class "TDMS datalogger configuration.lvclass">)
              n168 = property class="TDMS datalogger configuration"(reference=w313) -> (reference out=w311:refnum<class "TDMS datalogger configuration.lvclass">, error out=w310:errorcluster, "logrotate_options"=w312:T16)  [unwired: 1 in]
              n169 = Bundle By Name(cluster=w312, "No archive dir"="archive in place") -> (w309:T16)
              n170 = property class="TDMS datalogger configuration"(reference=w311, error in=w310, "logrotate_options"=w309) -> (reference out=w307:refnum<class "TDMS datalogger configuration.lvclass">, error out=w305:errorcluster)
              n171 = Compound Arithmetic op=AND(invert "archive in place", w301) -> (w304:bool)
              n172 = Compound Arithmetic op=AND(invert "archive in place", invert w301) -> (w303:bool)
              n173 = property on="Archive Directory" class="Str"("Visible"=w304) -> ()  [unwired: 2 in, 2 out]
              n174 = property on="Archive Directory" class="Path"("Visible"=w303) -> ()  [unwired: 2 in, 2 out]
              n175 = Bundle By Name(cluster=w308, "TDMS datalogger configuration"=w307) -> (w306:refnum<class "TDMS datalogger editor node.lvclass">)
              n176 = in-place-dvr #9(w306) -> (w298:errorcluster)  [unwired: 1 out]
            }
            n177 = Merge Errors(w298, w297) -> (w299:errorcluster)
          }
          event "Rotate count": Value Change {
            n178 = event-data() -> ()  [unwired: 1 in, 6 out]
            n179 = in-place {
              in-place-border: [w319] -> w315
              n180 = in-place-dvr #10(w317) -> (w322:refnum<class "TDMS datalogger editor node.lvclass">)  [unwired: 1 out]
              n181 = Unbundle By Name(w322) -> ("TDMS datalogger configuration"=w327:refnum<class "TDMS datalogger configuration.lvclass">)
              n182 = property class="TDMS datalogger configuration"(reference=w327) -> (reference out=w325:refnum<class "TDMS datalogger configuration.lvclass">, error out=w324:errorcluster, "logrotate_options"=w326:T16)  [unwired: 1 in]
              n183 = Bundle By Name(cluster=w326, "rotate count"="Rotate count") -> (w323:T16)
              n184 = property class="TDMS datalogger configuration"(reference=w325, error in=w324, "logrotate_options"=w323) -> (reference out=w321:refnum<class "TDMS datalogger configuration.lvclass">, error out=w319:errorcluster)
              n185 = Bundle By Name(cluster=w322, "TDMS datalogger configuration"=w321) -> (w320:refnum<class "TDMS datalogger editor node.lvclass">)
              n186 = in-place-dvr #10(w320) -> (w314:errorcluster)  [unwired: 1 out]
            }
            n187 = Merge Errors(w314, w315) -> (w316:errorcluster)
          }
          event "Maximum file size (KB)": Value Change {
            n188 = event-data() -> ()  [unwired: 1 in, 6 out]
            n189 = in-place {
              in-place-border: [w335] -> w329
              n190 = in-place-dvr #11(w331) -> (w338:refnum<class "TDMS datalogger editor node.lvclass">)  [unwired: 1 out]
              n191 = Unbundle By Name(w338) -> ("TDMS datalogger configuration"=w343:refnum<class "TDMS datalogger configuration.lvclass">)
              n192 = property class="TDMS datalogger configuration"(reference=w343) -> (reference out=w341:refnum<class "TDMS datalogger configuration.lvclass">, error out=w340:errorcluster, "logrotate_options"=w342:T16)  [unwired: 1 in]
              n193 = Multiply(x="Maximum file size (KB)", y=i64 1000) -> (x*y=w333:i64)
              n194 = Bundle By Name(cluster=w342, "max file size (bytes)"=w333) -> (w339:T16)
              n195 = property class="TDMS datalogger configuration"(reference=w341, error in=w340, "logrotate_options"=w339) -> (reference out=w337:refnum<class "TDMS datalogger configuration.lvclass">, error out=w335:errorcluster)
              n196 = Bundle By Name(cluster=w338, "TDMS datalogger configuration"=w337) -> (w336:refnum<class "TDMS datalogger editor node.lvclass">)
              n197 = in-place-dvr #11(w336) -> (w328:errorcluster)  [unwired: 1 out]
            }
            n198 = Merge Errors(w328, w329) -> (w330:errorcluster)
          }
          event "Maximum age of files (days)": Value Change {
            n199 = event-data() -> ()  [unwired: 1 in, 6 out]
            n200 = in-place {
              in-place-border: [w349] -> w345
              n201 = in-place-dvr #12(w347) -> (w352:refnum<class "TDMS datalogger editor node.lvclass">)  [unwired: 1 out]
              n202 = Unbundle By Name(w352) -> ("TDMS datalogger configuration"=w357:refnum<class "TDMS datalogger configuration.lvclass">)
              n203 = property class="TDMS datalogger configuration"(reference=w357) -> (reference out=w355:refnum<class "TDMS datalogger configuration.lvclass">, error out=w354:errorcluster, "logrotate_options"=w356:T16)  [unwired: 1 in]
              n204 = Bundle By Name(cluster=w356, "max age (days)"="Maximum age of files (days)") -> (w353:T16)
              n205 = property class="TDMS datalogger configuration"(reference=w355, error in=w354, "logrotate_options"=w353) -> (reference out=w351:refnum<class "TDMS datalogger configuration.lvclass">, error out=w349:errorcluster)
              n206 = Bundle By Name(cluster=w352, "TDMS datalogger configuration"=w351) -> (w350:refnum<class "TDMS datalogger editor node.lvclass">)
              n207 = in-place-dvr #12(w350) -> (w344:errorcluster)  [unwired: 1 out]
            }
            n208 = Merge Errors(w344, w345) -> (w346:errorcluster)
          }
          event "Enable Dynamic Mapping", "Channel Subscription Pattern Matches": Value Change {
            n209 = event-data() -> ()  [unwired: 1 in, 1 out]
            n210 = in-place {
              in-place-border: [w362] -> w361
              n211 = in-place-dvr #13(w359) -> (w371:refnum<class "TDMS datalogger editor node.lvclass">, w363:errorcluster)
              n212 = Unbundle By Name(w371) -> ("TDMS datalogger configuration"=w364:refnum<class "TDMS datalogger configuration.lvclass">)
              n213 = Select(t="Channel Subscription Pattern Matches", s="Enable Dynamic Mapping", f=string[] []) -> (s? t:f=w367:string[])
              n214 = for {
                tunnel: w367 -> [w375] mode=indexing
                tunnel: [w375] -> w366 mode=indexing if=w373
                n215 = Empty String/Path?(string/path=w375) -> (empty?=w374:bool)
                n216 = Not(x=w374) -> (.not. x?=w373:bool)
              }
              n217 = local write "Channel Subscription Pattern Matches"(w366) -> ()
              n218 = property class="TDMS datalogger configuration"(reference=w364, error in=w363, "Data Access:channel pattern matches"=w366) -> (reference out=w365:refnum<class "TDMS datalogger configuration.lvclass">, error out=w362:errorcluster)
              n219 = property on="Channel Subscription Pattern Matches" class="Arr (strict)"("Visible"="Enable Dynamic Mapping") -> ()  [unwired: 2 in, 2 out]
              n220 = Bundle By Name(cluster=w371, "TDMS datalogger configuration"=w365) -> (w372:refnum<class "TDMS datalogger editor node.lvclass">)
              n221 = in-place-dvr #13(w372) -> (w360:errorcluster)  [unwired: 1 out]
            }
            n222 = Merge Errors(w361, w360) -> (w358:errorcluster)
          }
          event "use enable channel": Value Change {
            n223 = event-data() -> ()  [unwired: 1 in, 1 out]
            n224 = Generate User Event(user event=w383, event data cluster=T14 {"command"="Refresh", "data"=""} ("event data")) -> ()  [unwired: 2 in, 2 out]
            n225 = in-place {
              in-place-border: [w400] -> w382
              in-place-border: [w394] -> w377
              n226 = in-place-dvr #14(w379) -> (w398:refnum<class "Engine Parent Editor Node.lvclass">, w396:errorcluster)
              n227 = in-place-dvr #15(w380) -> (w392:refnum<class "TDMS datalogger editor node.lvclass">, w395:errorcluster)
              n228 = Unbundle By Name(w392) -> ("TDMS datalogger configuration"=w393:refnum<class "TDMS datalogger configuration.lvclass">)
              n229 = call <vilib>:"read engine configuration.vi"("error in"=w396, "Engine Parent Editor Node in"=w398) -> ("error out"=w386:errorcluster, "engine configuration"=w397:refnum<class "engine configuration.lvclass">, "Engine Parent Editor Node out"=w388:refnum<class "Engine Parent Editor Node.lvclass">)  [unwired: 7 in]
              n230 = Merge Errors(w386, w395) -> (w385:errorcluster)
              n231 = case shown="True" "use enable channel" {
                tunnel: [w415 w436] -> w387
                tunnel: w397 -> [w418 w432]
                tunnel: [w420 w435] -> w402
                tunnel: w393 -> [w406 w425]
                tunnel: [w411 w430] -> w401
                tunnel: w385 -> [w408 w427]
                frame False {
                  n232 = call <vilib>:"Read UID.vi"("error in"=w408, "configuration in"=w406) -> ("error out"=w407:errorcluster, "instance id"=w405:string, "configuration out"=w404:refnum<class "TDMS datalogger configuration.lvclass">)  [unwired: 7 in]
                  n233 = call "create enable channel.vi"("error in"=w407, "TDMS datalogger configuration"=w404) -> ("error out"=w419:errorcluster, "enable channel name"=w403:string, "enable channel"=w417:refnum<class "TBM channel.lvclass">)  [unwired: 7 in]
                  n234 = call "remove channel from configuration.vi"("error in"=w419, "TBM channel in"=w417, "TDMS datalogger configuration in"=w404) -> ("error out"=w410:errorcluster, "TDMS datalogger configuration out"=w420:refnum<class "TDMS datalogger configuration.lvclass">)  [unwired: 7 in]
                  n235 = call <vilib>:"Clear Errors.vi"("error in (no error)"=w410) -> ("error out"=w409:errorcluster)  [unwired: 5 in, 1 out]
                  n236 = call <vilib>:"delete mapping by channel.vi"("owner ID"=w405, "error in"=w409, "channel"=w417, "engine configuration in"=w418) -> ("error out"=w413:errorcluster, "engine configuration out"=w416:refnum<class "engine configuration.lvclass">)  [unwired: 6 in]
                  n237 = call <vilib>:"Clear Errors.vi"("error in (no error)"=w413) -> ("error out"=w414:errorcluster)  [unwired: 5 in, 1 out]
                  n238 = call <vilib>:"delete tag.vi"("error in"=w414, "tag name"=w403, "engine configuration in"=w416) -> ("error out"=w412:errorcluster, "engine configuration out"=w415:refnum<class "engine configuration.lvclass">)  [unwired: 7 in]
                  n239 = call <vilib>:"Clear Errors.vi"("error in (no error)"=w412) -> ("error out"=w411:errorcluster)  [unwired: 5 in, 1 out]
                }
                frame True {
                  n240 = call <vilib>:"Read UID.vi"("error in"=w427, "configuration in"=w425) -> ("error out"=w426:errorcluster, "instance id"=w424:string, "configuration out"=w422:refnum<class "TDMS datalogger configuration.lvclass">)  [unwired: 7 in]
                  n241 = call "create enable channel.vi"("error in"=w426, "TDMS datalogger configuration"=w422) -> ("error out"=w434:errorcluster, "enable channel name"=→"Enable Tag":string, "enable channel"=w433:refnum<class "TBM channel.lvclass">)  [unwired: 7 in]
                  n242 = call "add channel to configuration.vi"("error in"=w434, "TBM channel in"=w433, "TDMS datalogger configuration in"=w422) -> ("error out"=w429:errorcluster, "TDMS datalogger configuration out"=w435:refnum<class "TDMS datalogger configuration.lvclass">)  [unwired: 7 in]
                  n243 = call <vilib>:"Clear Errors.vi"("error in (no error)"=w429) -> ("error out"=w428:errorcluster)  [unwired: 5 in, 1 out]
                  n244 = call <vilib>:"add and map fixed channel mapping.vi"("set module as owner"=FALSE, "module instance"=w424, "error in"=w428, "fixed channel"=w433, "engine configuration in"=w432) -> ("error out"=w431:errorcluster, "engine configuration out"=w436:refnum<class "engine configuration.lvclass">)  [unwired: 5 in]
                  n245 = call <vilib>:"Clear Errors.vi"("error in (no error)"=w431) -> ("error out"=w430:errorcluster)  [unwired: 5 in, 1 out]
                }
              }
              n246 = call "Write add enable channel.vi"("error in (no error)"=w401, "add enable channel"="use enable channel", "TDMS datalogger configuration in"=w402) -> ("error out"=w400:errorcluster, "TDMS datalogger configuration out"=w391:refnum<class "TDMS datalogger configuration.lvclass">)  [unwired: 7 in]
              n247 = Bundle By Name(cluster=w392, "TDMS datalogger configuration"=w391) -> (w390:refnum<class "TDMS datalogger editor node.lvclass">)
              n248 = call <vilib>:"write engine configuration.vi"("error in"=w386, "engine configuration"=w387, "Engine Parent Editor Node in"=w388) -> ("error out"=w394:errorcluster, "Engine Parent Editor Node out"=w389:refnum<class "Engine Parent Editor Node.lvclass">)  [unwired: 7 in]
              n249 = in-place-dvr #14(w389) -> (w378:errorcluster)  [unwired: 1 out]
              n250 = in-place-dvr #15(w390) -> (w376:errorcluster)  [unwired: 1 out]
            }
            n251 = Merge Errors(w382, w378, w377, w376) -> (w381:errorcluster)
          }
          event Value Change {
            n252 = event-data() -> ()  [unwired: 1 in, 1 out]
            n253 = Generate User Event(user event=w444, event data cluster=T14 {"command"="Refresh", "data"=""} ("event data")) -> ()  [unwired: 2 in, 2 out]
            n254 = in-place {
              in-place-border: [w449] -> w440
              in-place-border: [w458] -> w441
              n255 = in-place-dvr #16(w438) -> (w460:refnum<class "Engine Parent Editor Node.lvclass">, w461:errorcluster)
              n256 = in-place-dvr #17(w439) -> (w457:refnum<class "TDMS datalogger editor node.lvclass">, w463:errorcluster)
              n257 = call <vilib>:"read engine configuration.vi"("error in"=w461, "Engine Parent Editor Node in"=w460) -> ("error out"=w456:errorcluster, "engine configuration"=w447:refnum<class "engine configuration.lvclass">, "Engine Parent Editor Node out"=w459:refnum<class "Engine Parent Editor Node.lvclass">)  [unwired: 7 in]
              n258 = Unbundle By Name(w457) -> ("TDMS datalogger configuration"=w451:refnum<class "TDMS datalogger configuration.lvclass">)
              n259 = Merge Errors(w456, w463) -> (w446:errorcluster)
              n260 = local read "avail tags"() -> (w453:i32)
              n261 = property on="avail tags" class="MCListbox (strict)"(error in=w446) -> (error out=w454:errorcluster, "ItemNames"=w452:string[][])  [unwired: 1 in, 1 out]
              n262 = Index Array(array=w452, index (row)=w453) -> (element=w455:string[])  [unwired: 1 in]
              n263 = call "add tag by line.vi"("ItemNames"=w455, "error in"=w454, "TDMS datalogger configuration in"=w451, "engine configuration in"=w447) -> ("error out"=w449:errorcluster, "TDMS datalogger configuration out"=w450:refnum<class "TDMS datalogger configuration.lvclass">, "engine configuration out"=w448:refnum<class "engine configuration.lvclass">)  [unwired: 5 in]
              n264 = Bundle By Name(cluster=w457, "TDMS datalogger configuration"=w450) -> (w464:refnum<class "TDMS datalogger editor node.lvclass">)
              n265 = call <vilib>:"write engine configuration.vi"("error in"=w456, "engine configuration"=w448, "Engine Parent Editor Node in"=w459) -> ("error out"=w458:errorcluster, "Engine Parent Editor Node out"=w462:refnum<class "Engine Parent Editor Node.lvclass">)  [unwired: 7 in]
              n266 = in-place-dvr #16(w462) -> (w442:errorcluster)  [unwired: 1 out]
              n267 = in-place-dvr #17(w464) -> (w443:errorcluster)  [unwired: 1 out]
            }
            n268 = Merge Errors(w440, w442, w441, w443) -> (w437:errorcluster)
          }
          event Value Change {
            n269 = event-data() -> ()  [unwired: 1 in, 1 out]
            n270 = Generate User Event(user event=w472, event data cluster=T14 {"command"="Refresh", "data"=""} ("event data")) -> ()  [unwired: 2 in, 2 out]
            n271 = in-place {
              in-place-border: [w475] -> w471
              in-place-border: [w484] -> w470
              n272 = in-place-dvr #18(w465) -> (w486:refnum<class "Engine Parent Editor Node.lvclass">, w487:errorcluster)
              n273 = in-place-dvr #19(w466) -> (w483:refnum<class "TDMS datalogger editor node.lvclass">, w489:errorcluster)
              n274 = call <vilib>:"read engine configuration.vi"("error in"=w487, "Engine Parent Editor Node in"=w486) -> ("error out"=w482:errorcluster, "engine configuration"=w477:refnum<class "engine configuration.lvclass">, "Engine Parent Editor Node out"=w485:refnum<class "Engine Parent Editor Node.lvclass">)  [unwired: 7 in]
              n275 = Unbundle By Name(w483) -> ("TDMS datalogger configuration"=w478:refnum<class "TDMS datalogger configuration.lvclass">)
              n276 = Merge Errors(w482, w489) -> (w474:errorcluster)
              n277 = property on="avail tags" class="MCListbox (strict)"(error in=w474) -> (error out=w480:errorcluster, "ItemNames"=w481:string[][])  [unwired: 1 in, 1 out]
              n278 = for {
                tunnel: w481 -> [w491] mode=indexing
                shift-right: [w496] -> w475
                shift-left: w480 -> [w494]
                shift-right: [w497] -> w479
                shift-left: w478 -> [w495]
                shift-right: [w492] -> w476
                shift-left: w477 -> [w493]
                n279 = call "add tag by line.vi"("ItemNames"=w491, "error in"=w494, "TDMS datalogger configuration in"=w495, "engine configuration in"=w493) -> ("error out"=w496:errorcluster, "TDMS datalogger configuration out"=w497:refnum<class "TDMS datalogger configuration.lvclass">, "engine configuration out"=w492:refnum<class "engine configuration.lvclass">)  [unwired: 5 in]
              }
              n280 = Bundle By Name(cluster=w483, "TDMS datalogger configuration"=w479) -> (w490:refnum<class "TDMS datalogger editor node.lvclass">)
              n281 = call <vilib>:"write engine configuration.vi"("error in"=w482, "engine configuration"=w476, "Engine Parent Editor Node in"=w485) -> ("error out"=w484:errorcluster, "Engine Parent Editor Node out"=w488:refnum<class "Engine Parent Editor Node.lvclass">)  [unwired: 7 in]
              n282 = in-place-dvr #18(w488) -> (w469:errorcluster)  [unwired: 1 out]
              n283 = in-place-dvr #19(w490) -> (w468:errorcluster)  [unwired: 1 out]
            }
            n284 = Merge Errors(w471, w469, w470, w468) -> (w467:errorcluster)
          }
          event Value Change {
            n285 = event-data() -> ()  [unwired: 1 in, 1 out]
            n286 = local read "channels"() -> (w502:i32)
            n287 = Generate User Event(user event=w500, event data cluster=T14 {"command"="Refresh", "data"=""} ("event data")) -> ()  [unwired: 2 in, 2 out]
            n288 = case shown="0.." w502 {
              selector: w502 -> [_ w505]
              tunnel: [errorcluster {"status"=FALSE, "code"=0, "source"=""} ("error IO") w508] -> w503
              tunnel: w499 -> [_ w507]
              tunnel: w498 -> [_ w506]
              frame ..-1 {
              }
              frame 0.. {
                n289 = in-place {
                  in-place-border: [w521] -> w512
                  in-place-border: [w531] -> w511
                  in-place-border: w505 -> [w523]
                  n290 = in-place-dvr #20(w506) -> (w533:refnum<class "Engine Parent Editor Node.lvclass">, w534:errorcluster)
                  n291 = in-place-dvr #21(w507) -> (w530:refnum<class "TDMS datalogger editor node.lvclass">, w536:errorcluster)
                  n292 = call <vilib>:"read engine configuration.vi"("error in"=w534, "Engine Parent Editor Node in"=w533) -> ("error out"=w519:errorcluster, "engine configuration"=w522:refnum<class "engine configuration.lvclass">, "Engine Parent Editor Node out"=w532:refnum<class "Engine Parent Editor Node.lvclass">)  [unwired: 7 in]
                  n293 = Unbundle By Name(w530) -> ("TDMS datalogger configuration"=w517:refnum<class "TDMS datalogger configuration.lvclass">, "channel table"=w514:refnum<vi>)
                  n294 = Merge Errors(w519, w536) -> (w524:errorcluster)
                  n295 = property class="LstBox (strict)"(reference=w514) -> ("Item Names"=w513:string[])  [unwired: 1 in, 2 out]
                  n296 = call <vilib>:"Read UID.vi"("error in"=w524, "configuration in"=w517) -> ("error out"=w518:errorcluster, "instance id"=w515:string, "configuration out"=w516:refnum<class "TDMS datalogger configuration.lvclass">)  [unwired: 7 in]
                  n297 = Index Array(array=w513, index=w523) -> (element=w527:string)
                  n298 = call "find channel by name.vi"("channel name"=w527, "TDMS datalogger configuration in"=w516) -> ("channel"=w526:refnum<class "TBM channel.lvclass">, "TDMS datalogger configuration out"=w528:refnum<class "TDMS datalogger configuration.lvclass">)  [unwired: 8 in]
                  n299 = call "remove channel from configuration.vi"("error in"=w518, "TBM channel in"=w526, "TDMS datalogger configuration in"=w528) -> ("error out"=w529:errorcluster, "TDMS datalogger configuration out"=w525:refnum<class "TDMS datalogger configuration.lvclass">)  [unwired: 7 in]
                  n300 = call <vilib>:"delete mapping by channel.vi"("owner ID"=w515, "error in"=w529, "channel"=w526, "engine configuration in"=w522) -> ("error out"=w521:errorcluster, "engine configuration out"=w520:refnum<class "engine configuration.lvclass">)  [unwired: 6 in]
                  n301 = Bundle By Name(cluster=w530, "TDMS datalogger configuration"=w525) -> (w537:refnum<class "TDMS datalogger editor node.lvclass">)
                  n302 = call <vilib>:"write engine configuration.vi"("error in"=w519, "engine configuration"=w520, "Engine Parent Editor Node in"=w532) -> ("error out"=w531:errorcluster, "Engine Parent Editor Node out"=w535:refnum<class "Engine Parent Editor Node.lvclass">)  [unwired: 7 in]
                  n303 = in-place-dvr #20(w535) -> (w510:errorcluster)  [unwired: 1 out]
                  n304 = in-place-dvr #21(w537) -> (w509:errorcluster)  [unwired: 1 out]
                }
                n305 = Merge Errors(w512, w510, w511, w509) -> (w508:errorcluster)
              }
            }
          }
          event Value Change {
            n306 = event-data() -> ()  [unwired: 1 in, 1 out]
            n307 = Generate User Event(user event=w543, event data cluster=T14 {"command"="Refresh", "data"=""} ("event data")) -> ()  [unwired: 2 in, 2 out]
            n308 = in-place {
              in-place-border: "Logging Type" -> [w550]
              in-place-border: [w551] -> w541
              n309 = in-place-dvr #22(w542) -> (w556:refnum<class "TDMS datalogger editor node.lvclass">, w553:errorcluster)
              n310 = Unbundle By Name(w556) -> ("TDMS datalogger configuration"=w557:refnum<class "TDMS datalogger configuration.lvclass">)
              n311 = local read "Total Blocks to Log"() -> (w545:i32)
              n312 = Equal?(x=w550, y=Logging_Type."Continuous") -> (x = y?=w548:bool)
              n313 = Select(t=-1 ("Value (Signaling)"), s=w548, f=w545) -> (s? t:f=w546:i32)
              n314 = property class="TDMS datalogger configuration"(reference=w557, error in=w553, "Logging Type"=w550) -> (reference out=w554:refnum<class "TDMS datalogger configuration.lvclass">, error out=w552:errorcluster)
              n315 = Bundle By Name(cluster=w556, "TDMS datalogger configuration"=w554) -> (w555:refnum<class "TDMS datalogger editor node.lvclass">)
              n316 = property on="Total Blocks to Log" class="DigNum (strict)"(error in=w552, "Val(Sgnl)"=w546) -> (error out=w551:errorcluster)  [unwired: 1 in, 1 out]
              n317 = in-place-dvr #22(w555) -> (w539:errorcluster)  [unwired: 1 out]
            }
            n318 = Merge Errors(w539, w541) -> (w540:errorcluster)
          }
          event Value Change {
            n319 = event-data() -> ()  [unwired: 1 in, 6 out]
            n320 = in-place {
              in-place-border: "Edge Direction" -> [w568]
              in-place-border: [w563] -> w561
              n321 = in-place-dvr #23(w562) -> (w567:refnum<class "TDMS datalogger editor node.lvclass">, w564:errorcluster)
              n322 = Unbundle By Name(w567) -> ("TDMS datalogger configuration"=w569:refnum<class "TDMS datalogger configuration.lvclass">)
              n323 = property class="TDMS datalogger configuration"(reference=w569, error in=w564, "Data Access:Edge Direction"=w568) -> (reference out=w565:refnum<class "TDMS datalogger configuration.lvclass">, error out=w563:errorcluster)
              n324 = Bundle By Name(cluster=w567, "TDMS datalogger configuration"=w565) -> (w566:refnum<class "TDMS datalogger editor node.lvclass">)
              n325 = in-place-dvr #23(w566) -> (w559:errorcluster)  [unwired: 1 out]
            }
            n326 = Merge Errors(w559, w561) -> (w560:errorcluster)
          }
          event Value Change {
            n327 = event-data() -> ()  [unwired: 1 in, 6 out]
            n328 = Generate User Event(user event=w578, event data cluster=T14 {"command"="Refresh", "data"=""} ("event data")) -> (error out=w573:errorcluster)  [unwired: 2 in, 1 out]
            n329 = in-place {
              in-place-border: w573 -> [w599]
              in-place-border: [w587] -> w574
              in-place-border: [w593] -> w575
              n330 = in-place-dvr #24(w570) -> (w594:refnum<class "Engine Parent Editor Node.lvclass">, w595:errorcluster)
              n331 = in-place-dvr #25(w571) -> (w592:refnum<class "TDMS datalogger editor node.lvclass">, w597:errorcluster)
              n332 = call <vilib>:"read engine configuration.vi"("error in"=w595, "Engine Parent Editor Node in"=w594) -> ("error out"=w591:errorcluster, "engine configuration"=w589:refnum<class "engine configuration.lvclass">, "Engine Parent Editor Node out"=w590:refnum<class "Engine Parent Editor Node.lvclass">)  [unwired: 7 in]
              n333 = Unbundle By Name(w592) -> ("TDMS datalogger configuration"=w581:refnum<class "TDMS datalogger configuration.lvclass">)
              n334 = Merge Errors(w599, w591, w597) -> (w583:errorcluster)
              n335 = property class="TDMS datalogger configuration"(reference=w581, error in=w583, "Data Access:Trigger Type"="Trigger Type") -> (reference out=w580:refnum<class "TDMS datalogger configuration.lvclass">, error out=w584:errorcluster)
              n336 = call "Handle Trigger Channel.vi"("error in (no error)"=w584, "Trigger Type"="Trigger Type", "TDMS datalogger configuration"=w580, "engine configuration in"=w589) -> ("error out"=w587:errorcluster, "trigger channel name"=→"Trigger Channel":string, "TDMS datalogger configuration out"=w586:refnum<class "TDMS datalogger configuration.lvclass">, "engine configuration out"=w588:refnum<class "engine configuration.lvclass">)  [unwired: 4 in]
              n337 = Bundle By Name(cluster=w592, "TDMS datalogger configuration"=w586) -> (w598:refnum<class "TDMS datalogger editor node.lvclass">)
              n338 = call <vilib>:"write engine configuration.vi"("error in"=w591, "engine configuration"=w588, "Engine Parent Editor Node in"=w590) -> ("error out"=w593:errorcluster, "Engine Parent Editor Node out"=w596:refnum<class "Engine Parent Editor Node.lvclass">)  [unwired: 7 in]
              n339 = in-place-dvr #24(w596) -> (w576:errorcluster)  [unwired: 1 out]
              n340 = in-place-dvr #25(w598) -> (w577:errorcluster)  [unwired: 1 out]
            }
            n341 = Merge Errors(w574, w576, w575, w577) -> (w572:errorcluster)
          }
          event "Filter": Value Change {
            n342 = event-data() -> ()  [unwired: 1 in, 1 out]
            n343 = global read "Table Items.vi" "Channels"() -> (w600:string[])
            n344 = call "Apply filter.vi"("Filter"="Filter", "Item names"=w600) -> ("Filtered Item Names"=w607:string[])  [unwired: 9 in]
            n345 = property on="channels" class="LstBox (strict)"(error in=w603, "Item Names"=w607) -> (error out=w601:errorcluster)  [unwired: 1 in, 1 out]
            n346 = global read "Table Items.vi" "Available Tags"() -> (w602:string[][])
            n347 = for {
              tunnel: w602 -> [w609] mode=indexing
              tunnel: "Filter" -> [w610]
              tunnel: [w609] -> w605 mode=indexing if=w608
              n348 = Index Array(array=w609) -> (element=w611:string)  [unwired: 1 in]
              n349 = Match Pattern(string=w611, regular expression=w610) -> (offset past match=w612:i32)  [unwired: 1 in, 3 out]
              n350 = Greater Or Equal To 0?(x=w612) -> (x >= 0?=w608:bool)
            }
            n351 = property on="avail tags" class="MCListbox (strict)"(error in=w601, "ItemNames"=w605) -> (error out=w604:errorcluster)  [unwired: 1 in, 1 out]
          }
        }
        n352 = case shown="Error" w117 {
          selector: w117 -> [w120 w124]
          tunnel: [w121 w125] -> w116
          tunnel: w111 -> [w121 w125]
          tunnel: [w120 w122] -> w115
          frame No Error {
          }
          frame Error {
            # "#CodeRecommended Any errors should be handled within the generating case or here. Current default is to clear everything"
            n353 = call <vilib>:"Simple Error Handler.vi"("error in (no error)"=w124) -> ("error out"=w123:errorcluster)  [unwired: 4 in, 4 out]
            n354 = call <vilib>:"Clear Errors.vi"("error in (no error)"=w123) -> ("error out"=w122:errorcluster)  [unwired: 5 in, 1 out]
          }
        }
      }
    }
    frame Error {
    }
  }
  n355 = disable-structure shown="Disabled" {
    frame Disabled {
      n356 = in-place {
        in-place-border: _ -> [w628]
        in-place-border: [_] -> w615
        in-place-border: [w621] -> w616
        n357 = in-place-dvr #26() -> (w623:refnum<class "Engine Parent Editor Node.lvclass">, w624:errorcluster)  [unwired: 1 in]
        n358 = in-place-dvr #27() -> (w620:refnum<class "TDMS datalogger editor node.lvclass">, w626:errorcluster)  [unwired: 1 in]
        n359 = call <vilib>:"read engine configuration.vi"("error in"=w624, "Engine Parent Editor Node in"=w623) -> ("error out"=w619:errorcluster, "Engine Parent Editor Node out"=w622:refnum<class "Engine Parent Editor Node.lvclass">)  [unwired: 7 in, 1 out]
        n360 = Unbundle By Name(w620) -> ()  [unwired: 1 out]
        n361 = Merge Errors(w628, w619, w626) -> ()  [unwired: 1 out]
        n362 = Bundle By Name(cluster=w620) -> (w627:refnum<class "TDMS datalogger editor node.lvclass">)  [unwired: 1 in]
        n363 = call <vilib>:"write engine configuration.vi"("error in"=w619, "Engine Parent Editor Node in"=w622) -> ("error out"=w621:errorcluster, "Engine Parent Editor Node out"=w625:refnum<class "Engine Parent Editor Node.lvclass">)  [unwired: 8 in]
        n364 = in-place-dvr #26(w625) -> (w617:errorcluster)  [unwired: 1 out]
        n365 = in-place-dvr #27(w627) -> (w618:errorcluster)  [unwired: 1 out]
      }
      n366 = Merge Errors(w615, w617, w616, w618) -> ()  [unwired: 1 out]
    }
    frame Enabled {
    }
  }
  n367 = Unregister For Events(event registration refnum=w60, error in=w41) -> (error out=w59:errorcluster)
  n368 = call <vilib>:"Simple Error Handler.vi"("error in (no error)"=w59) -> ()  [unwired: 4 in, 5 out]
